vi "Class_Find All Matches.vi"(4 "Groups To Find":refnum<class>, 5 "GroupList":refnum<class>[](array[class])) -> (1 "Classes Found Out":refnum<class>[](array[class]))   [LabVIEW 2015]
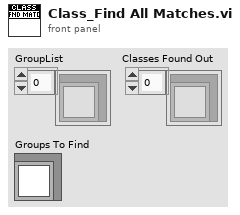
[diagram p1: front panel]
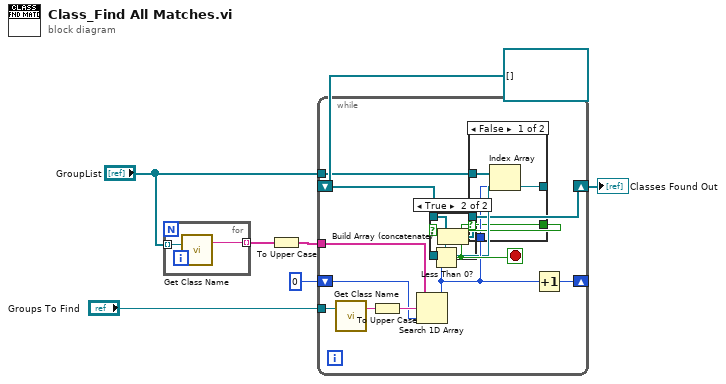
[diagram p0: block diagram]
diagram:
  n1 = for {
    tunnel: "GroupList" -> [w9] mode=indexing
    tunnel: [w8] -> w7 mode=indexing
    n2 = call "Get Class Name.vi"("lvclass"=w9) -> ("Child Name"=w8:string)  [unwired: 3 in, 1 out]
  }
  n3 = To Upper Case(1:w7) -> (0:w6:string[])
  n4 = while {
    tunnel: w6 -> [w22]
    tunnel: "Groups To Find" -> [w21]
    shift-right: [w17] -> _
    shift-left: 0 -> [w18]
    tunnel: "GroupList" -> [w15]
    shift-right: [w10] -> w2
    shift-left: refnum<class>[] [] ("Array") -> [w11]
    stop <- w16 stop-if-true
    n5 = call "Get Class Name.vi"("lvclass"=w21) -> ("Child Name"=w20:string)  [unwired: 3 in, 1 out]
    n6 = To Upper Case(1:w20) -> (0:w19:string)
    n7 = Search 1D Array(1D array=w22, element=w19, start index (0)=w18) -> (index of element=w14:i32)
    n8 = Less Than 0?(x=w14) -> (x < 0?=w16:bool)
    n9 = case shown="False" w16 {
      selector: w16 -> [w27 _]
      tunnel: w15 -> [w30 _]
      tunnel: w14 -> [w29 _]
      tunnel: [w28 _] -> w13
      tunnel: [w27 _] -> w12
      frame False {
        n10 = Index Array(array=w30, index=w29) -> (element=w28:refnum<class>)
      }
      frame True {
      }
    }
    n11 = case shown="True" w12 {
      tunnel: w11 -> [w23 w25]
      tunnel: w13 -> [_ w24]
      tunnel: [w23 w26] -> w10
      frame False {
      }
      frame True {
        n12 = Build Array (concatenate)(w25, w24) -> (w26:refnum<class>[])
      }
    }
    n13 = Increment(x=w14) -> (x+1=w17:i32)
  }
  "Classes Found Out" <- w2
